vi "Center Pane.vi"(8 "error in (no error)":errorcluster) -> (0 "error out":errorcluster)   [LabVIEW 2017]
uses:
  <vilib>/Utility/miscctls.llb/LVPointTypeDef.ctl
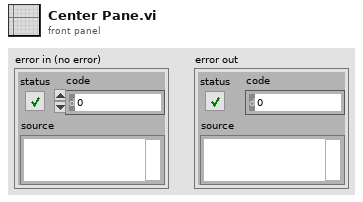
[diagram p1: front panel]
types:
  T1 = typedef "LVPointTypeDef.ctl" = cluster{"Horizontal":i16, "Vertical":i16}
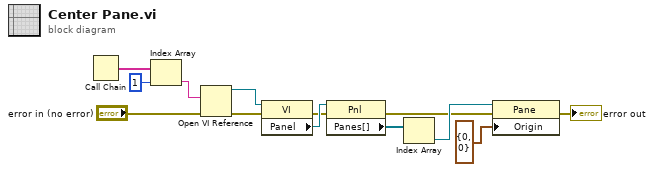
[diagram p0: block diagram]
diagram:
  n1 = Call Chain() -> (call chain=w4:string[])
  n2 = Index Array(array=w4, index=1) -> (element=w6:string)
  n3 = Open VI Reference(vi path=w6, error in (no error)="error in (no error)") -> (vi reference=w3:refnum<vi>, error out=w1:errorcluster)  [unwired: 4 in]
  n4 = property class="VI"(reference=w3, error in=w1) -> (error out=w9:errorcluster, "Panel"=w12:refnum<vi>)  [unwired: 1 out]
  n5 = property class="Pnl"(reference=w12, error in=w9) -> (error out=w8:errorcluster, "Panes[]"=w11:refnum<vi>[])  [unwired: 1 out]
  n6 = Index Array(array=w11) -> (element=w10:refnum<vi>)  [unwired: 1 in]
  n7 = property on="Property Node" class="Pane"(reference=w10, error in=w8, "Origin"=T1 {"Horizontal"=0, "Vertical"=0}) -> (error out=→"error out":errorcluster)  [unwired: 1 out]
